vi "SetDigitalOutput.vi"(4 "error in (no error)":errorcluster, 5 "active state":bool, 6 "digital output configuration":u16(ring) items=["ready/fault"=0, "position compare"=1, "general purpose A"=15, "general purpose B"=14, "general purpose C"=13, "general purpose D"=12, "general purpose E"=11, "general purpose F"=10, "general purpose G"=9, "general purpose H"=8], 7 "axis in":cluster{"keyHandle":u32, "nodeId":u16}={"keyHandle"=0, "nodeId"=1}) -> (0 "error out":errorcluster, 3 "axis out":cluster{"keyHandle":u32, "nodeId":u16}={"keyHandle"=0, "nodeId"=1})   [LabVIEW 2018]
doc: "<B>SetDigitalOutput</B> changes one digital output state in the device."
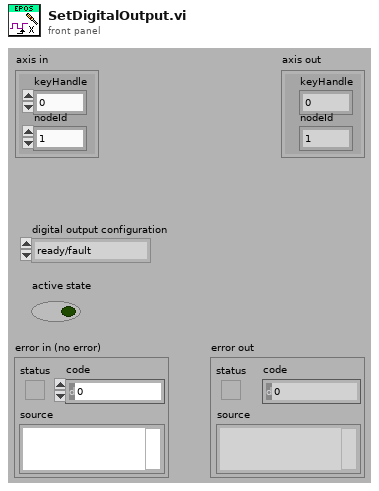
[diagram p1: front panel]
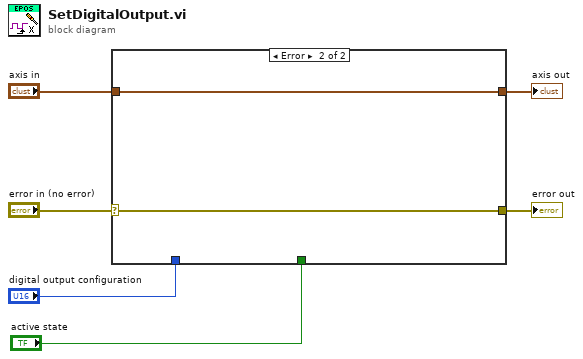
[diagram p0: block diagram]
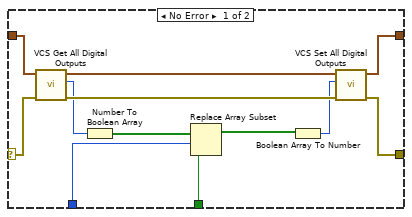
[diagram p2: hidden frame]
diagram:
  n1 = case shown="Error" "error in (no error)" {
    selector: "error in (no error)" -> [w17 w20]
    tunnel: [w15 w20] -> w5
    tunnel: [w14 w19] -> w4
    tunnel: "axis in" -> [w18 w19]
    tunnel: "digital output configuration" -> [w8 _]
    tunnel: "active state" -> [w7 _]
    frame No Error {
      n2 = call "VCS Get All Digital Outputs.vi"("error in (no error)"=w17, "axis in"=w18) -> ("error out"=w16:errorcluster, "digitalOutputs"=w12:u16, "axis out"=w13:cluster{"keyHandle":u32, "nodeId":u16})  [unwired: 7 in]
      n3 = Number To Boolean Array(number=w12) -> (Boolean array=w10:bool[])
      n4 = Replace Array Subset(array=w10, new element=w7, index=w8) -> (w9:bool[])
      n5 = Boolean Array To Number(Boolean array=w9) -> (number=w11:u32)
      n6 = call "VCS Set All Digital Outputs.vi"("error in (no error)"=w16, "outputs"=w11, "axis in"=w13) -> ("error out"=w15:errorcluster, "axis out"=w14:cluster{"keyHandle":u32, "nodeId":u16})  [unwired: 7 in]
    }
    frame Error {
    }
  }
  "error out" <- w5
  "axis out" <- w4
